vi "FPGA_MAIN_lock-in.vi"() -> ()   [LabVIEW 2010]
uses:
  <vilib>/eio/EIONode/EIONode.xnode
  <vilib>/rvi/eio/nirviEIOImplementation/nirviEIOImplementation.xnode
  <vilib>/rvi/eio/common/nirviEmuClasses.ctl
  <vilib>/rvi/DataTransferAndStorage/Container/XNode/niFpgaContainer.xnode
  <vilib>/rvi/eio/common/nirviEmuTemplateMethod_noerrors.vi
  <vilib>/rvi/FIFO/Fifo_Resource/nirvififoEmulationSetSize.vi
  <vilib>/rvi/DataTransferAndStorage/Container/Common/niFpgaContainerGetUniqueNameForEmu.vi
  <vilib>/rvi/Memory/Memory_Emulation/nirvimemoryEmulationManagerCache_GetValue.vi
  <vilib>/rvi/Memory/Memory_Emulation/nirvimemoryEmulationManagerCache_InsertValue.vi
  <vilib>/Utility/error.llb/Clear Errors.vi
  <vilib>/rvi/Memory/Memory_Emulation/nirvimemoryEmulationManagerCache_SetValue.vi
panel:
  in  "DAC to retrieve":u16
  in  "got DAC value":bool
  out "DAC data":u32
  out "get DAC value":bool
  out "move bus ready":bool=TRUE
  out "sending order":bool
  out "subsystem":u8
  in  "order in":u64
  in  "order Xmitted":bool
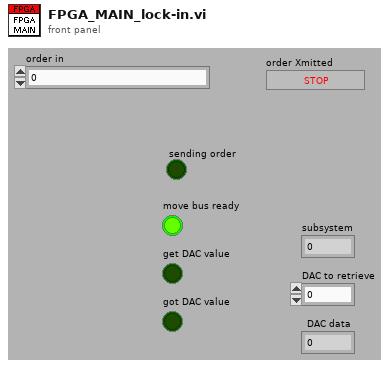
[diagram p1: front panel]
types:
  T1 = typedef "nirviEmuClasses.ctl" = enum16{"IO Read", "IO Write", "Method", "Property Read", "Property Write"}
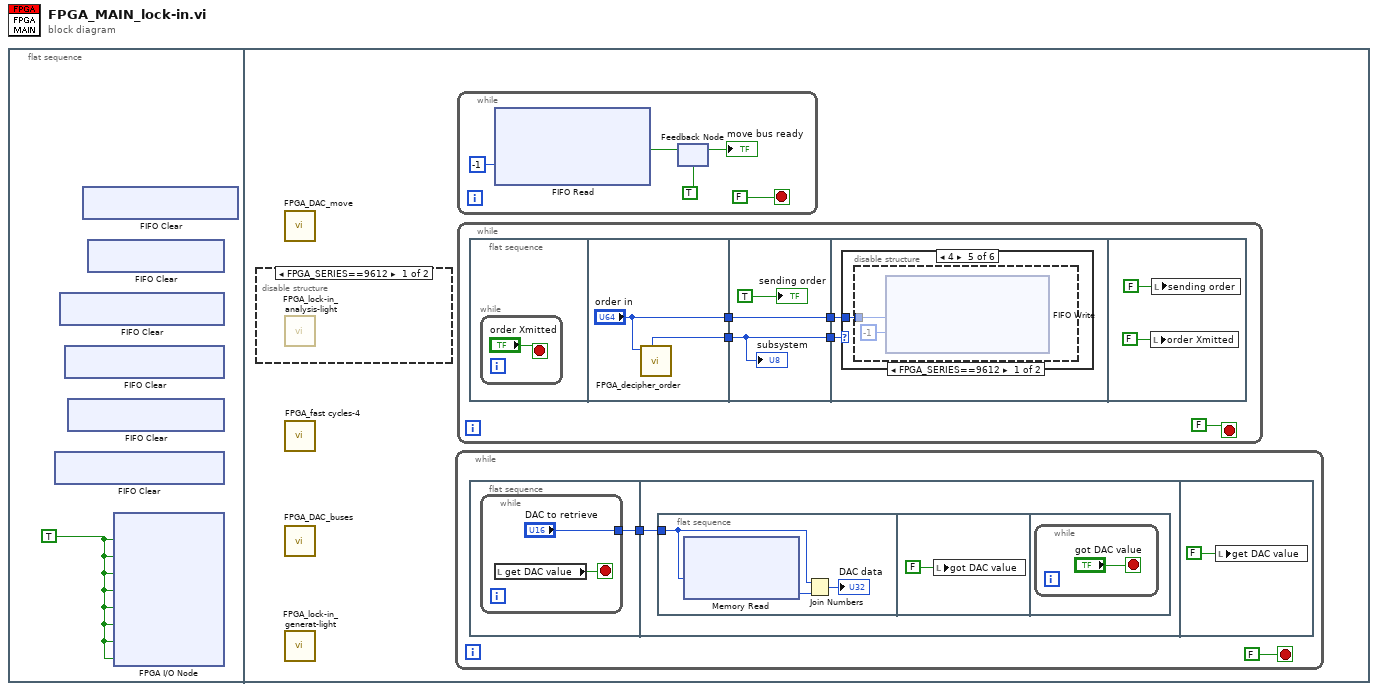
[diagram p0: block diagram]
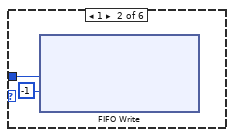
[diagram p4: hidden frame]
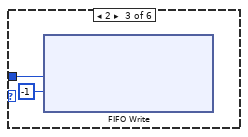
[diagram p5: hidden frame]
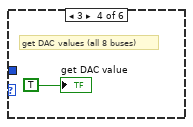
[diagram p6: hidden frame]
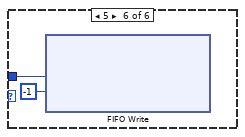
[diagram p8: hidden frame]
diagram:
  n1 = flat-sequence {
    frame #0 {
      w1 = TRUE ("Port0/DIOCTL")
      n2 = xnode ("FIFO Clear")() -> ()  [unwired: 1 in, 1 out]
      n3 = xnode ("FIFO Clear")() -> ()  [unwired: 1 in, 1 out]
      n4 = xnode ("FIFO Clear")() -> ()  [unwired: 1 in, 1 out]
      n5 = xnode ("FIFO Clear")() -> ()  [unwired: 1 in, 1 out]
      n6 = xnode ("FIFO Clear")() -> ()  [unwired: 1 in, 1 out]
      n7 = xnode ("FIFO Clear")() -> ()  [unwired: 1 in, 1 out]
      n8 = xnode "FPGA I/O Node"("Port0/DIOCTL"=w1, "Port1/DIOCTL"=w1, "Port2/DIOCTL"=w1, "Port3/DIOCTL"=w1, "Port4/DIOCTL"=w1, "Port5/DIOCTL"=w1, "Port6/DIOCTL"=w1, "Port7/DIOCTL"=w1) -> ()  [unwired: 8 in, 8 out]
    }
    frame #1 {
      n9 = disable-structure shown="FPGA_SERIES==9612" {
        frame condition #0 {
          n10 = call "FPGA_lock-in_analysis-light.vi"() -> ()  [unwired: 1 out]
        }
        frame condition #1 (active) {
        }
      }
      n11 = call "FPGA_DAC_move.vi"() -> ()  [unwired: 12 out]
      n12 = call "FPGA_fast cycles-4.vi"() -> ()  [unwired: 1 out]
      n13 = call "FPGA_DAC_buses.vi"() -> ()  [unwired: 12 out]
      n14 = call "FPGA_lock-in_generat-light.vi"() -> ()  [unwired: 1 out]
      n15 = while {
        stop <- FALSE stop-if-true
        n16 = flat-sequence {
          tunnel: [w326] -> w324
          tunnel: w324 -> [w329]
          frame #0 {
            n17 = while {
              tunnel: ["DAC to retrieve"] -> w326
              stop <- w328 stop-if-true
              n18 = local read "get DAC value"() -> (w328:bool)
            }
          }
          frame #1 {
            n19 = flat-sequence {
              tunnel: w329 -> [w330]
              frame #0 {
                n20 = xnode ("Memory Read")("Address"=w330) -> ("Data"=w332:u16)  [unwired: 1 in, 1 out]
                n21 = Join Numbers(hi=w330, lo=w332) -> ((hi.lo)=→"DAC data":u32)
              }
              frame #1 {
                n22 = local write "got DAC value"(FALSE ("got DAC value")) -> ()
              }
              frame #2 {
                n23 = while {
                  stop <- "got DAC value" stop-if-true
                }
              }
            }
          }
          frame #2 {
            n24 = local write "get DAC value"(FALSE ("get DAC values")) -> ()
          }
        }
      }
      n25 = while {
        stop <- FALSE stop-if-true
        n26 = xnode ("FIFO Read")("Timeout"=-1) -> ("Element"=w465:bool)  [unwired: 1 in, 2 out]
        n27 = feedback-in #1(w465) -> ()
        n28 = feedback #1(TRUE ("Element")) -> (→"move bus ready":bool)
      }
      n29 = while {
        stop <- FALSE stop-if-true
        n30 = flat-sequence {
          tunnel: [w525] -> w520
          tunnel: ["order in"] -> w519
          tunnel: [w528] -> w521
          tunnel: w520 -> [w528]
          tunnel: w519 -> [w526]
          tunnel: [w526] -> w518
          tunnel: w521 -> [w530]
          tunnel: w518 -> [w529]
          frame #0 {
            n31 = while {
              stop <- "order Xmitted" stop-if-true
            }
          }
          frame #1 {
            n32 = call "FPGA_decipher_order.vi"("order in"="order in") -> ("subsystem"=w525:u8)  [unwired: 10 out]
          }
          frame #2 {
            "sending order" <- TRUE ("Boolean")
            "subsystem" <- w528
          }
          frame #3 {
            n33 = case shown="4" w530 {
              tunnel: w529 -> [_ w531 w584 _ w638 w692]
              frame 0, Default {
              }
              frame 1 {
                n34 = xnode ("FIFO Write")("Element"=w531, "Timeout"=-1) -> ()  [unwired: 1 in, 2 out]
              }
              frame 2 {
                n35 = xnode ("FIFO Write")("Element"=w584, "Timeout"=-1) -> ()  [unwired: 1 in, 2 out]
              }
              frame 3 {
                # "get DAC values (all 8 buses)"
                "get DAC value" <- TRUE ("get DAC values")
              }
              frame 4 {
                n36 = disable-structure shown="FPGA_SERIES==9612" {
                  disable-tunnel: w638 -> [w640 _]
                  frame condition #0 {
                    n37 = xnode ("FIFO Write")("Element"=w640, "Timeout"=-1) -> ()  [unwired: 1 in, 2 out]
                  }
                  frame condition #1 (active) {
                  }
                }
              }
              frame 5 {
                n38 = xnode ("FIFO Write")("Element"=w692, "Timeout"=-1) -> ()  [unwired: 1 in, 2 out]
              }
            }
          }
          frame #4 {
            n39 = local write "order Xmitted"(FALSE ("order Xmitted")) -> ()
            n40 = local write "sending order"(FALSE ("sending order")) -> ()
          }
        }
      }
    }
  }
